vi "configure relay.vi"(8 "error in":errorcluster, 11 "Node Ref in":T1) -> (0 "error out":errorcluster, 1 "Event Reg Ref":refnum<event-registration>, 3 "Node Ref out":T1)   [LabVIEW 2023, in "Publisher Subscriber.lvlib"]
uses:
  <userlib>/_Publisher Subscriber/Publisher Subscriber.lvlib
  <userlib>/_Publisher Subscriber/Controls/data cluster.ctl
  <userlib>/_Publisher Subscriber/Controls/node refnum.ctl
  <userlib>/_Publisher Subscriber/Controls/node dvr data.ctl
  <userlib>/_Publisher Subscriber/Controls/subscription bank ref.ctl
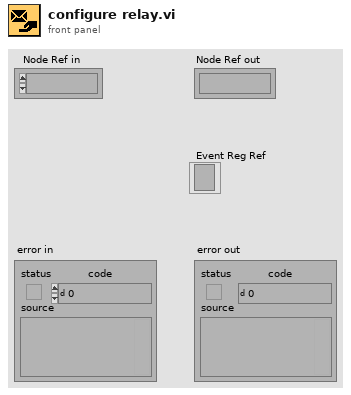
[diagram p1: front panel]
types:
  T1 = typedef "Publisher Subscriber.lvlib/node refnum.ctl" = refnum<vi>
  T2 = typedef "Publisher Subscriber.lvlib/data cluster.ctl" = cluster{"Command":string, "Data":variant}
  T3 = typedef "Publisher Subscriber.lvlib/node dvr data.ctl" = cluster{"queue ref":refnum<queue>, "Subscription Bank Ref":refnum<data-value>, "Command":string, "Data":variant, "Subscriptions []":set{string}, "Variables DVR Ref":refnum<data-value>}
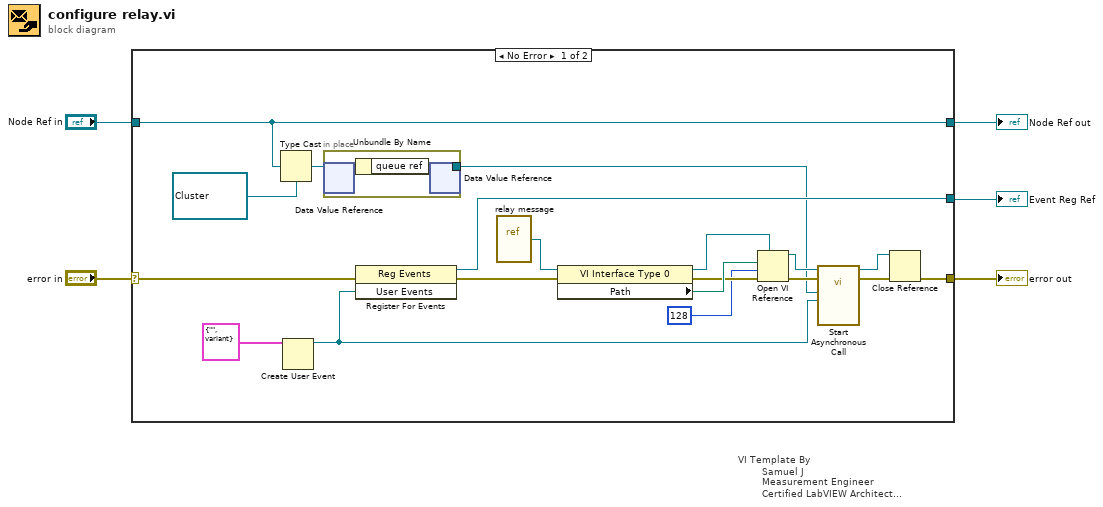
[diagram p0: block diagram]
diagram:
  n1 = case "VI Template By\n        Samuel J\n        Measurement Engineer\n        Certified LabVIEW Architect\n        Vestas Technology R&D Chennai" shown="No Error" "error in" {
    selector: "error in" -> [w13 w28]
    tunnel: [w12 w28] -> w4
    tunnel: [w10 _] -> w3
    tunnel: [w6 w27] -> w2
    tunnel: "Node Ref in" -> [w6 w27]
    frame No Error {
      n2 = Type Cast(type=refnum<data-value> refnum ("data value reference"), x=w6) -> (*(type *) &x=w8:refnum<data-value>)
      n3 = Create User Event(user event datatype=T2 {"Command"="", "Data"=variant} ("User Events")) -> (user event=w11:refnum<user-event>)  [unwired: 1 in, 1 out]
      n4 = in-place {
        in-place-border: [w25] -> w7
        n5 = in-place-dvr #1(w8) -> (w26:T3)  [unwired: 1 out]
        n6 = Unbundle By Name(w26) -> ("queue ref"=w25:refnum<queue>)
        n7 = in-place-dvr #1() -> ()  [unwired: 1 in, 2 out]
      }
      n8 = register-events(error in=w13, w11) -> (reference out=w10:refnum<event-registration>, error out=w24:errorcluster)  [unwired: 1 in]
      n9 = vi-ref <userlib>:"relay message.vi"() -> (w16:refnum<vi>)
      n10 = property class="VI Interface Type 0"(reference=w16, error in=w24) -> (reference out=w22:refnum<vi>, error out=w19:errorcluster, "Path"=w23:path)
      n11 = Open VI Reference(type specifier VI Refnum (for type only)=w22, vi path=w23, options=128, error in (no error)=w19) -> (vi reference=w17:refnum<vi>, error out=w20:errorcluster)  [unwired: 2 in]
      n12 = call-by-ref "Start Asynchronous Call"(reference=w17, error in=w20, "User Events"=w11, "queue ref"=w7) -> (reference out=w18:refnum<vi>, error out=w21:errorcluster)  [unwired: 10 in]
      n13 = Close Reference(reference=w18, error in (no error)=w21) -> (error out=w12:errorcluster)
    }
    frame Error {
    }
  }
  "Event Reg Ref" <- w3
  "Node Ref out" <- w2
  "error out" <- w4
